vi "GW_Cylinder_Up.vi"(7 "位置(記錄用)":string="790", 8 "error in (no error)":errorcluster, 9 "禁止覆蓋":bool, 10 "glue_id":i16, 11 "DBLink":string) -> (0 "error out":errorcluster, 2 "當前資料":string)   [LabVIEW 2019]
panel:
  # "此id位置為汽缸剛頂起，需搬移資料至此欄位"
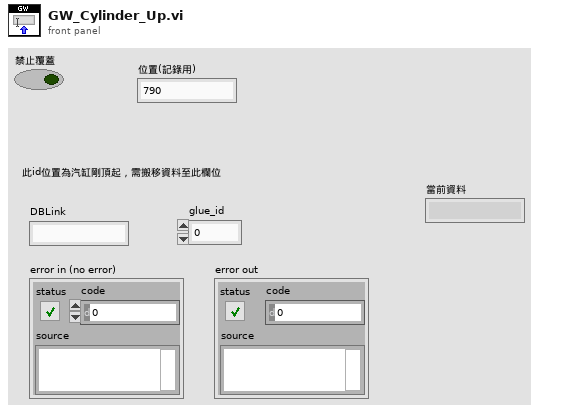
[diagram p1: front panel]
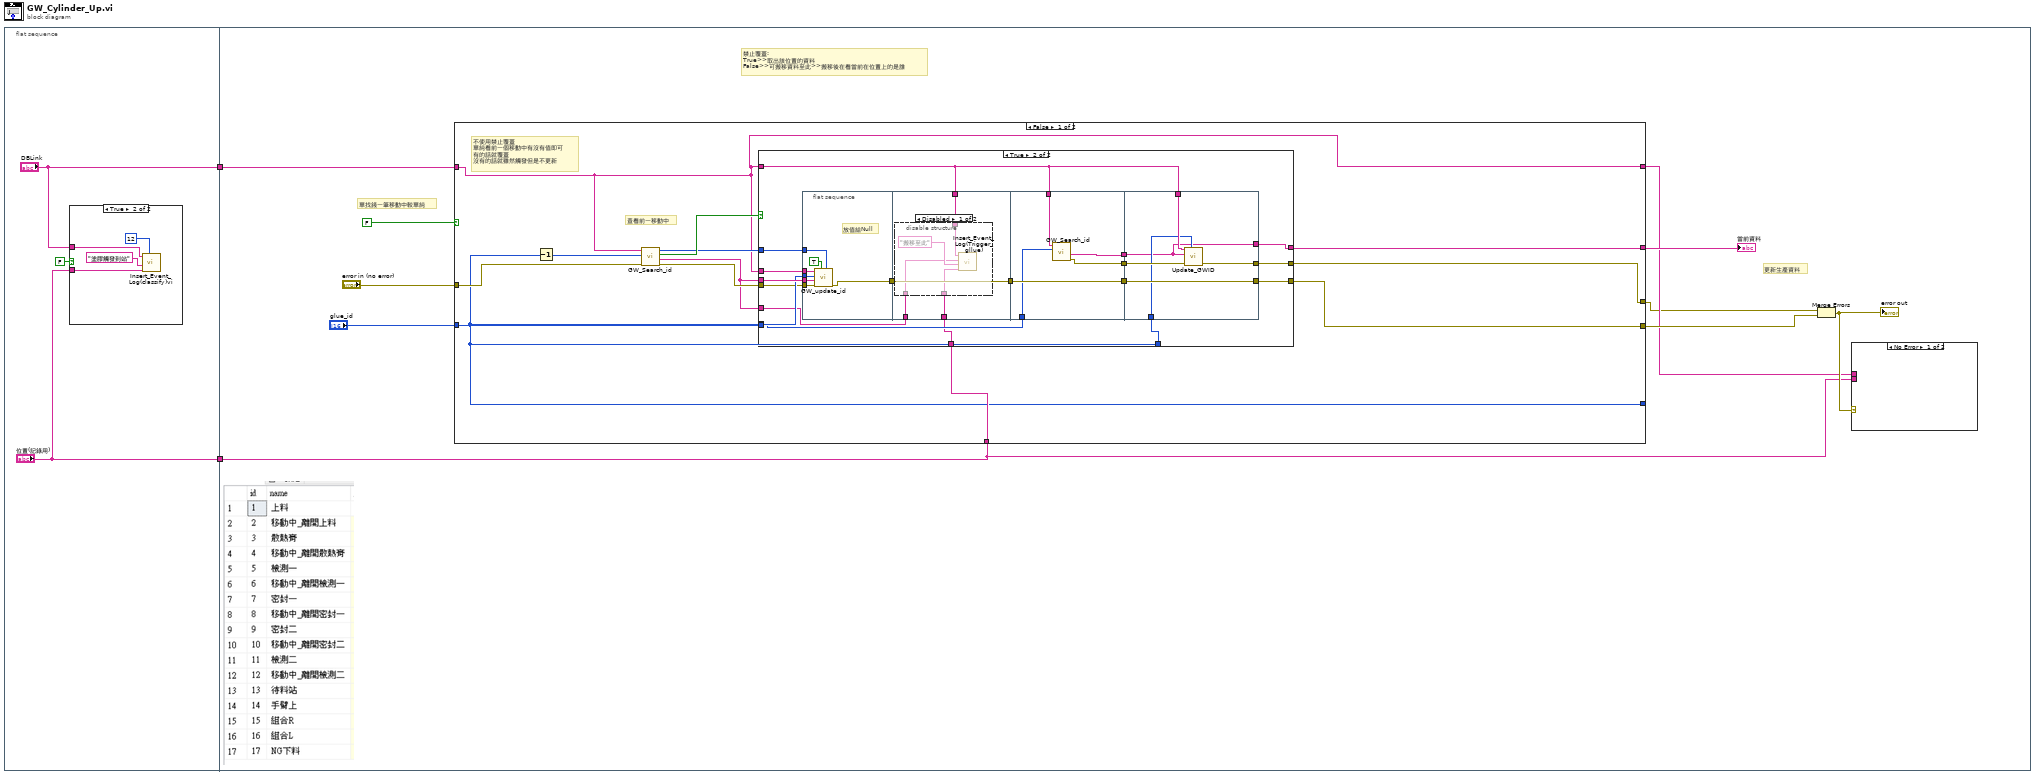
[diagram p0: block diagram]
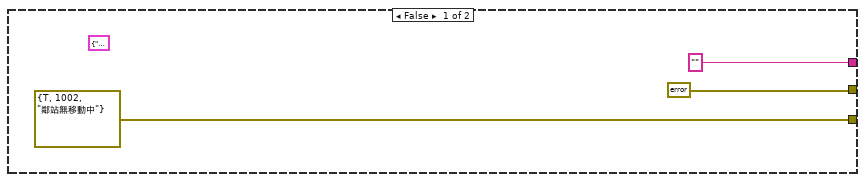
[diagram p3: hidden frame]
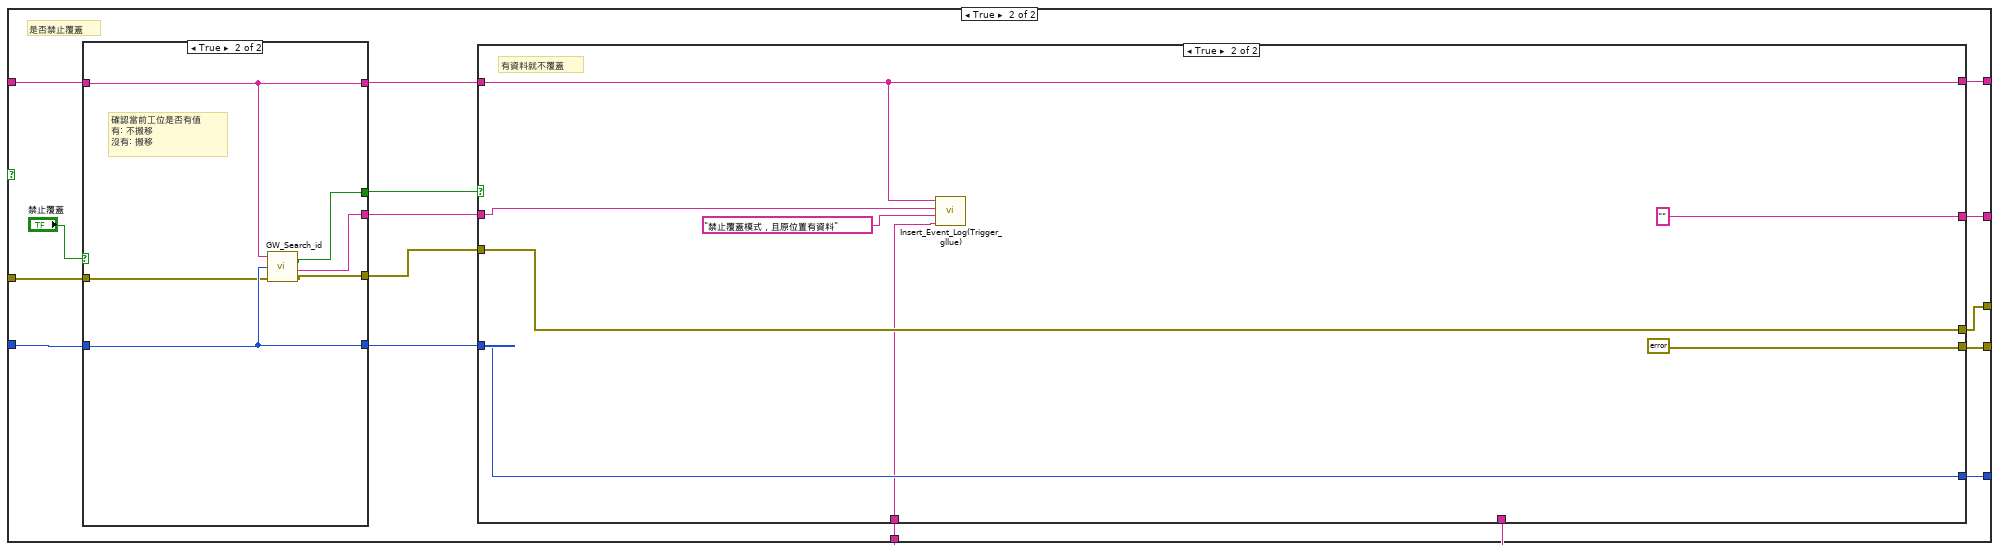
[diagram p5: hidden frame]
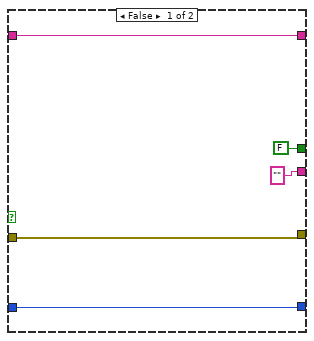
[diagram p6: hidden frame]
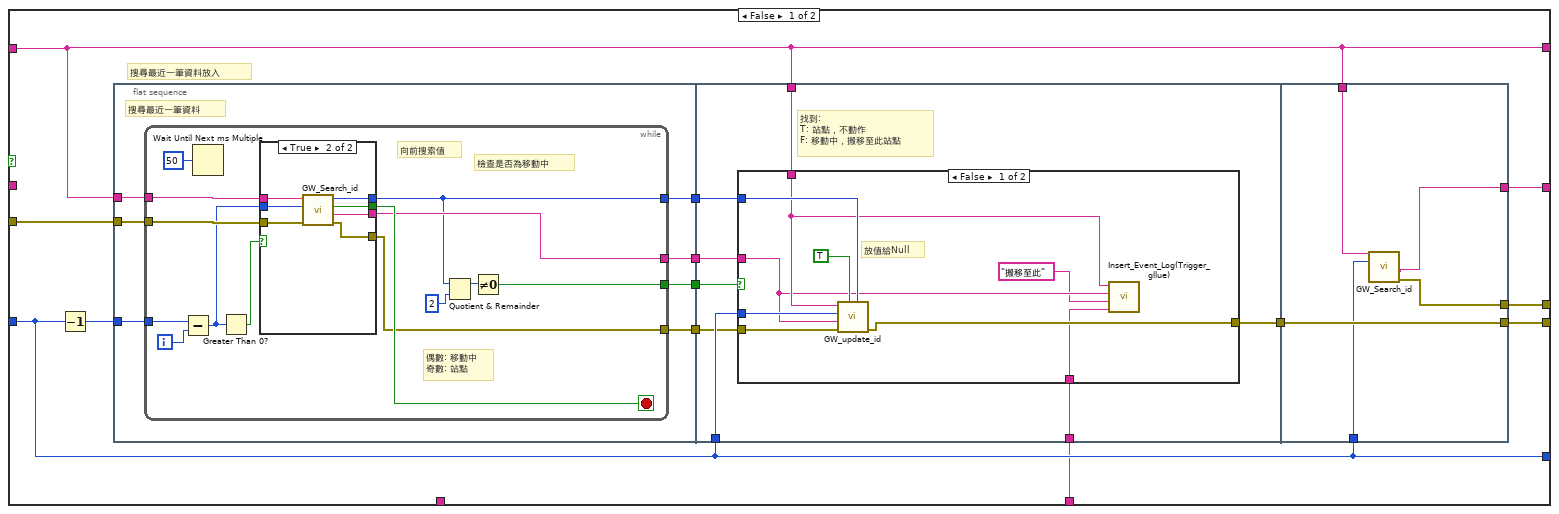
[diagram p7: hidden frame]
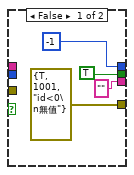
[diagram p8: hidden frame]
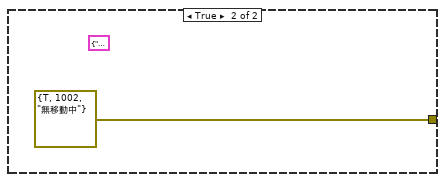
[diagram p9: hidden frame]
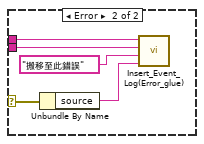
[diagram p10: hidden frame]
diagram:
  n1 = flat-sequence {
    tunnel: ["DBLink"] -> w2
    tunnel: ["位置(記錄用)"] -> w1
    tunnel: w2 -> [w12]
    tunnel: w1 -> [w11]
    frame #0 {
      n2 = case shown="True" FALSE {
        tunnel: "DBLink" -> [_ w7]
        tunnel: "位置(記錄用)" -> [_ w6]
        frame False {
        }
        frame True {
          n3 = call "Insert_Event_Log(classify)vi.vi"("classify"=i16 12, "data"=w6, "message"="塗膠觸發到站", "DBlink"=w7) -> ()  [unwired: 7 in, 1 out]
        }
      }
    }
    frame #1 {
      # "單找錢一筆移動中較單純"
      # "更新生產資料"
      # "禁止覆蓋:\nTrue>>取出該位置的資料\nFalse>>可搬移資料至此>>搬移後在看當前在位置上的是誰"
      n4 = case shown="False" FALSE {
        tunnel: w12 -> [w23 w93]
        tunnel: "error in (no error)" -> [w30 w92]
        tunnel: "glue_id" -> [w20 w91]
        tunnel: [w24 w86] -> w17
        tunnel: [w22 w84] -> w10
        tunnel: [w21 w83] -> w16
        tunnel: [w20 w82] -> _
        tunnel: [w23 w81] -> w14
        tunnel: w11 -> [w25 w80]
        frame False {
          # "查看前一移動中"
          # "不使用禁止覆蓋\n單純看前一個移動中有沒有值即可\n有的話就覆蓋\n沒有的話就雖然觸發但是不更新"
          n5 = Decrement(x=w20) -> (x-1=w31:i16)
          n6 = call "GW_Search_id.vi"("error in (no error)"=w30, "id"=w31, "DBlink"=w23) -> ("error out"=w27:errorcluster, "[glue_data_id]"=w26:string, "找到"=w29:bool, "取得ID"=w28:i16)  [unwired: 5 in]
          n7 = case shown="True" w29 {
            tunnel: [errorcluster {"status"=TRUE, "code"=1002, "source"="鄰站無移動中"} ("error constant") w52] -> w24
            tunnel: w23 -> [_ w51]
            tunnel: w26 -> [_ w50]
            tunnel: w20 -> [_ w49]
            tunnel: w28 -> [_ w48]
            tunnel: w27 -> [_ w47]
            tunnel: w26 -> [_ w42]
            tunnel: w23 -> [_ w37]
            tunnel: w25 -> [_ w41]
            tunnel: w20 -> [_ w46]
            tunnel: [errorcluster {"status"=FALSE, "code"=0, "source"=""} ("error out") w45] -> w22
            tunnel: ["" ("[glue_data_id]") w35] -> w21
            tunnel: w20 -> [_ w36]
            frame False {
              (unwired) cluster{"條碼R":string, "條碼L":string} {"條碼R"="", "條碼L"=""} ("workplace_data")
            }
            frame True {
              n8 = flat-sequence {
                tunnel: w51 -> [w57]
                tunnel: w50 -> [w56]
                tunnel: w49 -> [w55]
                tunnel: w48 -> [w54]
                tunnel: w47 -> [w53]
                tunnel: [w58] -> w44
                tunnel: w44 -> [w63]
                tunnel: [w63] -> w43
                tunnel: w42 -> [w62]
                tunnel: w41 -> [w61]
                tunnel: w37 -> [w60]
                tunnel: w43 -> [w72]
                tunnel: w46 -> [w71]
                tunnel: w37 -> [w68]
                tunnel: [w72] -> w40
                tunnel: [w70] -> w39
                tunnel: [w69] -> w38
                tunnel: [w74] -> w45
                tunnel: [w78] -> w52
                tunnel: w40 -> [w78]
                tunnel: w39 -> [w76]
                tunnel: w38 -> [w73]
                tunnel: w37 -> [w77]
                tunnel: w36 -> [w75]
                tunnel: [w73] -> w35
                frame #0 {
                  # "放值給Null"
                  n9 = call "GW_update_id.vi"("NULL: workplace_id"=w54, "Set null"=TRUE, "error in (no error)"=w53, "glue_data_id"=w56, "id"=w55, "DBlink"=w57) -> ("error out"=w58:errorcluster)  [unwired: 5 in]
                }
                frame #1 {
                  n10 = disable-structure shown="Disabled" {
                    disable-tunnel: w62 -> [w66 _]
                    disable-tunnel: w61 -> [w65 _]
                    disable-tunnel: w60 -> [w64 _]
                    frame Disabled {
                      n11 = call "Insert_Event_Log(Trigger_gllue).vi"("data"=w65, "message"="搬移至此", "id"=w66, "DBlink"=w64) -> ()  [unwired: 8 in]
                    }
                    frame Enabled {
                    }
                  }
                }
                frame #2 {
                  n12 = call "GW_Search_id.vi"("id"=w71, "DBlink"=w68) -> ("error out"=w70:errorcluster, "[glue_data_id]"=w69:string)  [unwired: 6 in, 2 out]
                }
                frame #3 {
                  n13 = call "Update_GWID .vi"("[glue_workspace_id]"=w75, "error in (no error)"=w76, "[glue_data_id]"=w73, "DBlink"=w77) -> ("error out"=w74:errorcluster)  [unwired: 7 in]
                }
              }
            }
          }
        }
        frame True {
          # "是否禁止覆蓋"
          n14 = case shown="True" "禁止覆蓋" {
            tunnel: w93 -> [w95 w104]
            tunnel: w92 -> [w98 w102]
            tunnel: w91 -> [w97 w103]
            tunnel: [w97 w103] -> w90
            tunnel: [w95 w104] -> w89
            tunnel: [FALSE ("找到") w101] -> w88
            tunnel: [w98 w100] -> w87
            tunnel: ["" ("條碼R") w99] -> w85
            frame False {
            }
            frame True {
              # "確認當前工位是否有值\n有: 不搬移\n沒有: 搬移"
              n15 = call "GW_Search_id.vi"("error in (no error)"=w102, "id"=w103, "DBlink"=w104) -> ("error out"=w100:errorcluster, "[glue_data_id]"=w99:string, "找到"=w101:bool)  [unwired: 5 in, 1 out]
            }
          }
          n16 = case shown="True" w88 {
            tunnel: w87 -> [w117 w180]
            tunnel: w90 -> [w110 w179]
            tunnel: w89 -> [w113 w177]
            tunnel: [w111 w180] -> w84
            tunnel: [w112 "" ("[glue_data_id]")] -> w83
            tunnel: [w113 w177] -> w81
            tunnel: [w110 w179] -> w82
            tunnel: [w106 errorcluster {"status"=FALSE, "code"=0, "source"=""} ("error constant")] -> w86
            tunnel: w85 -> [_ w176]
            tunnel: w80 -> [_ w174]
            tunnel: w80 -> [w105 _]
            frame False {
              # "搜尋最近一筆資料放入"
              n17 = Decrement(x=w110) -> (x-1=w116:i16)
              n18 = flat-sequence {
                tunnel: w113 -> [w124]
                tunnel: w117 -> [w123]
                tunnel: w116 -> [w122]
                tunnel: [w121] -> w115
                tunnel: [w120] -> w114
                tunnel: [w119] -> w109
                tunnel: [w118] -> w108
                tunnel: w115 -> [w157]
                tunnel: w113 -> [w156]
                tunnel: w110 -> [w155]
                tunnel: w114 -> [w154]
                tunnel: w109 -> [w153]
                tunnel: w108 -> [w152]
                tunnel: [w151] -> w107
                tunnel: w105 -> [w150]
                tunnel: w113 -> [w171]
                tunnel: w110 -> [w170]
                tunnel: [w169] -> w112
                tunnel: [w168] -> w111
                tunnel: w107 -> [w172]
                tunnel: [w172] -> w106
                frame #0 {
                  # "搜尋最近一筆資料"
                  n19 = while {
                    tunnel: w124 -> [w138]
                    tunnel: w123 -> [w136]
                    tunnel: w122 -> [w133]
                    tunnel: [w130] -> w121
                    tunnel: [w129] -> w120
                    tunnel: [w126] -> w119
                    tunnel: [w125] -> w118
                    i -> [w137]
                    stop <- w132 stop-if-true
                    # "偶數: 移動中\n奇數: 站點"
                    # "檢查是否為移動中"
                    # "向前搜索值"
                    n20 = Subtract(x=w133, y=w137) -> (x-y=w131:i32)
                    n21 = Wait Until Next ms Multiple(millisecond multiple=u32 50) -> ()  [unwired: 1 out]
                    n22 = Greater Than 0?(x=w131) -> (x > 0?=w135:bool)
                    n23 = case shown="True" w135 {
                      tunnel: w138 -> [_ w149]
                      tunnel: w136 -> [_ w147]
                      tunnel: [errorcluster {"status"=TRUE, "code"=1001, "source"="id<0\n無值"} ("error out") w146] -> w129
                      tunnel: w131 -> [_ w148]
                      tunnel: [TRUE ("找到") w144] -> w132
                      tunnel: [i16 -1 ("取得ID") w143] -> w125
                      tunnel: ["" ("[glue_data_id]") w145] -> w130
                      frame False {
                      }
                      frame True {
                        n24 = call "GW_Search_id.vi"("error in (no error)"=w147, "id"=w148, "DBlink"=w149) -> ("error out"=w146:errorcluster, "[glue_data_id]"=w145:string, "找到"=w144:bool, "取得ID"=w143:i16)  [unwired: 5 in]
                      }
                    }
                    n25 = Quotient & Remainder(x=w125, y=2) -> (x-y*floor(x/y)=w128:i32)  [unwired: 1 out]
                    n26 = Not Equal To 0?(x=w128) -> (x != 0?=w126:bool)
                  }
                }
                frame #1 {
                  # "找到: \nT: 站點，不動作\nF: 移動中，搬移至此站點"
                  n27 = case shown="False" w153 {
                    tunnel: [w162 errorcluster {"status"=TRUE, "code"=1002, "source"="無移動中"} ("error constant")] -> w151
                    tunnel: w157 -> [w160 _]
                    tunnel: w156 -> [w161 _]
                    tunnel: w155 -> [w166 _]
                    tunnel: w154 -> [w165 _]
                    tunnel: w152 -> [w163 _]
                    tunnel: w150 -> [w158 _]
                    frame False {
                      # "放值給Null"
                      n28 = call "GW_update_id.vi"("NULL: workplace_id"=w163, "Set null"=TRUE, "error in (no error)"=w165, "glue_data_id"=w160, "id"=w166, "DBlink"=w161) -> ("error out"=w162:errorcluster)  [unwired: 5 in]
                      n29 = call "Insert_Event_Log(Trigger_gllue).vi"("data"=w158, "message"="搬移至此", "id"=w160, "DBlink"=w161) -> ()  [unwired: 8 in]
                    }
                    frame True {
                      (unwired) cluster{"條碼R":string, "條碼L":string} {"條碼R"="", "條碼L"=""} ("workplace_data")
                    }
                  }
                }
                frame #2 {
                  n30 = call "GW_Search_id.vi"("id"=w170, "DBlink"=w171) -> ("error out"=w168:errorcluster, "[glue_data_id]"=w169:string)  [unwired: 6 in, 2 out]
                }
              }
            }
            frame True {
              # "有資料就不覆蓋"
              n31 = call "Insert_Event_Log(Trigger_gllue).vi"("data"=w174, "message"="禁止覆蓋模式，且原位置有資料", "id"=w176, "DBlink"=w177) -> ()  [unwired: 8 in]
            }
          }
        }
      }
      "當前資料" <- w16
      n32 = Merge Errors(w10, w17) -> (w15:errorcluster)
      "error out" <- w15
      n33 = case shown="No Error" w15 {
        selector: w15 -> [_ w182]
        tunnel: w14 -> [_ w185]
        tunnel: w11 -> [_ w183]
        frame No Error {
        }
        frame Error {
          n34 = Unbundle By Name(w182) -> ("source"=w181:string)
          n35 = call "Insert_Event_Log(Error_glue).vi"("data"=w181, "message"="搬移至此錯誤", "id"=w183, "DBlink"=w185) -> ()  [unwired: 8 in]
        }
      }
    }
  }
